vi "GetVersion.vi"(0 "controller in":refnum<k24>, 11 "error in (no error)":errorcluster) -> (4 "controller out":refnum<k24>, 6 "firmware version":string, 8 "fpga version":i32, 10 "hardware version":i32, 15 "error out":errorcluster)   [LabVIEW 2010]
uses:
  c:/aerotech/controller/5.xx.xxx/ensemble/pc/labview/2010/bin/Aerotech.Ensemble.dll
  bin/Aerotech.Ensemble.dll
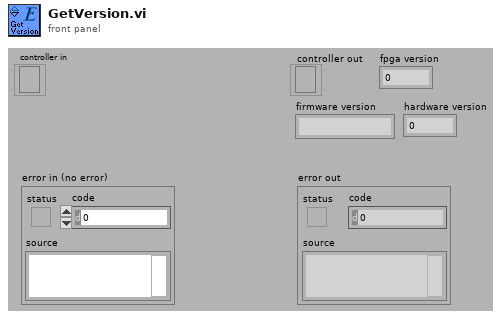
[diagram p1: front panel]
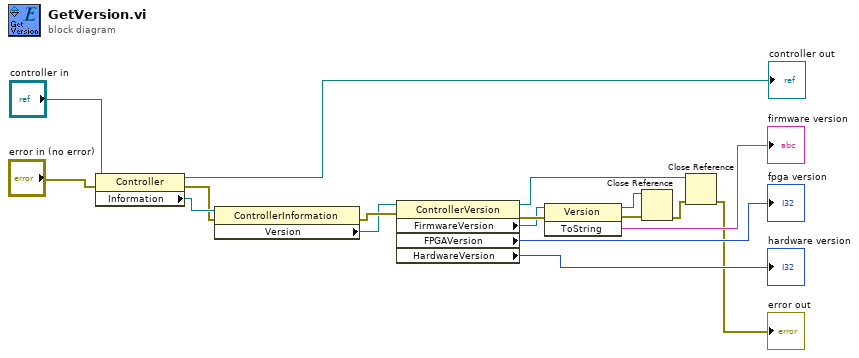
[diagram p0: block diagram]
diagram:
  n1 = property class="Controller"(reference="controller in", error in="error in (no error)") -> (reference out=→"controller out":refnum<k24>, error out=w3:errorcluster, "Information"=w7:refnum<k24>)
  n2 = property class="ControllerInformation"(reference=w7, error in=w3) -> (error out=w2:errorcluster, "Version"=w1:refnum<k24>)  [unwired: 1 out]
  n3 = property class="ControllerVersion"(reference=w1, error in=w2) -> (reference out=w10:refnum<k24>, error out=w14:errorcluster, "FirmwareVersion"=w8:refnum<k24>, "FPGAVersion"=→"fpga version":i32, "HardwareVersion"=→"hardware version":i32)
  n4 = invoke class="Version" method="ToString"(reference=w8, error in=w14) -> (reference out=w4:refnum<k24>, error out=w6:errorcluster, "ToString"=→"firmware version":string)  [unwired: 1 in]
  n5 = Close Reference(reference=w4, error in (no error)=w6) -> (error out=w5:errorcluster)
  n6 = Close Reference(reference=w10, error in (no error)=w5) -> (error out=→"error out":errorcluster)
